vi "caseStructure.vi"() -> ()   [LabVIEW 2021]
panel:
  out "Numeric":dbl
  in  "Boolean 2":bool
  out "s? t:f":dbl
  in  "Boolean":bool
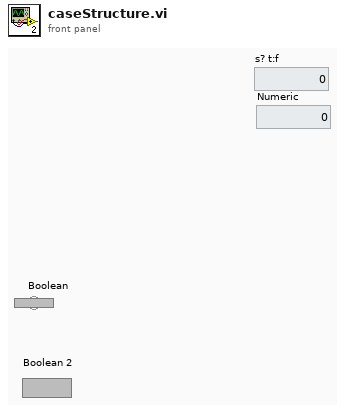
[diagram p1: front panel]
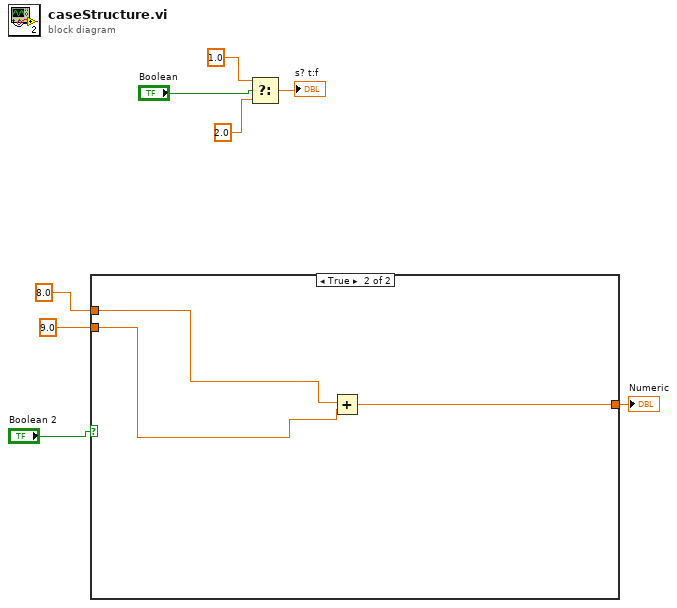
[diagram p0: block diagram]
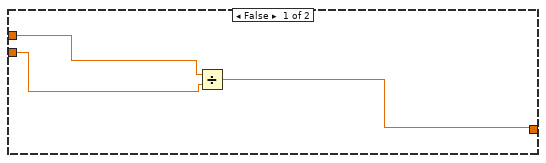
[diagram p2: hidden frame]
diagram:
  n1 = case shown="True" "Boolean 2" {
    tunnel: 9.0 -> [w10 w13]
    tunnel: 8.0 -> [w11 w14]
    tunnel: [w9 w12] -> w1
    frame False {
      n2 = Divide(x=w11, y=w10) -> (x/y=w9:dbl)
    }
    frame True {
      n3 = Add(x=w14, y=w13) -> (x+y=w12:dbl)
    }
  }
  "Numeric" <- w1
  n4 = Select(t=1.0, s="Boolean", f=2.0) -> (s? t:f=→"s? t:f":dbl)
